vi "FolderSkeleton.vi"() -> ()   [LabVIEW 2017]
panel:
  in  "Base Path":path=path "c:/ni-rt/LabVIEW Data/MyDataFolder1"
  in  "Folders Per Folder":i32=10
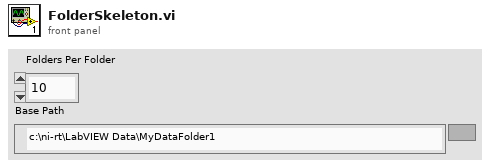
[diagram p1: front panel]
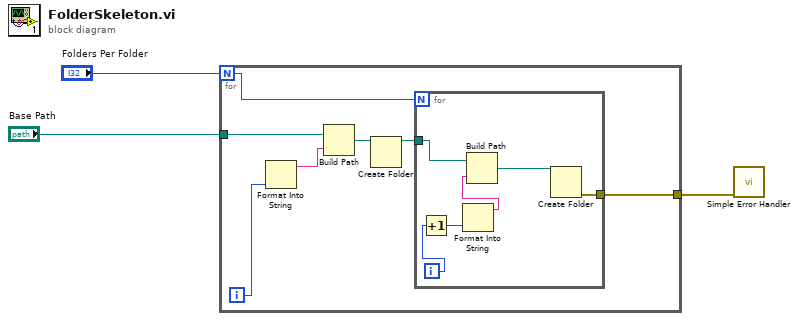
[diagram p0: block diagram]
diagram:
  n1 = for {
    N: "Folders Per Folder" -> [w5]
    tunnel: "Base Path" -> [w10]
    tunnel: [w4] -> w1
    i -> [w8]
    n2 = Format Into String(w8) -> (resulting string=w7:string)  [unwired: 3 in, 1 out]
    n3 = Build Path(base path=w10, name or relative path=w7) -> (appended path=w9:path)
    n4 = Create Folder(path (use dialog)=w9) -> (created path=w6:path)  [unwired: 2 in, 2 out]
    n5 = for {
      N: w5 -> [_]
      tunnel: w6 -> [w16]
      tunnel: [w11] -> w4
      i -> [w15]
      n6 = Increment(x=w15) -> (x+1=w14:i32)
      n7 = Format Into String(w14) -> (resulting string=w13:string)  [unwired: 3 in, 1 out]
      n8 = Build Path(base path=w16, name or relative path=w13) -> (appended path=w12:path)
      n9 = Create Folder(path (use dialog)=w12) -> (error out=w11:errorcluster)  [unwired: 2 in, 2 out]
    }
  }
  n10 = call <vilib>:"Simple Error Handler.vi"("error in (no error)"=w1) -> ()  [unwired: 4 in, 5 out]
